vi "Read Voltage.vi"(6 "错误输入":cluster{"状态":bool, "代码":i32, "源":string}) -> (0 "错误输出":cluster{"状态":bool, "代码":i32, "源":string}, 3 "电压":dbl)   [LabVIEW 2012]
doc: "该VI用于LabVIEW核心课程I、II。\n\n该VI可模拟从DAQ板卡获取电压读数。在本课程中，该VI可代替温度读数相关练习中的“DAQ助手”Express VI。该VI可作为所有（演示）练习中的子VI使用。"
panel:
  # "该VI可用于演示读取设备1上通道0的电压值。该值调整100倍后转换为温度值。"
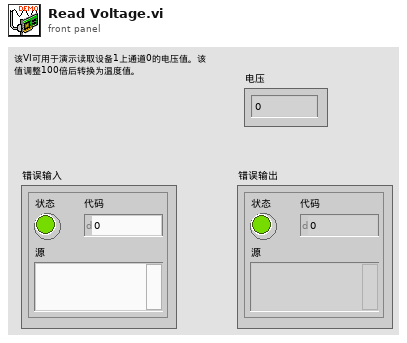
[diagram p1: front panel]
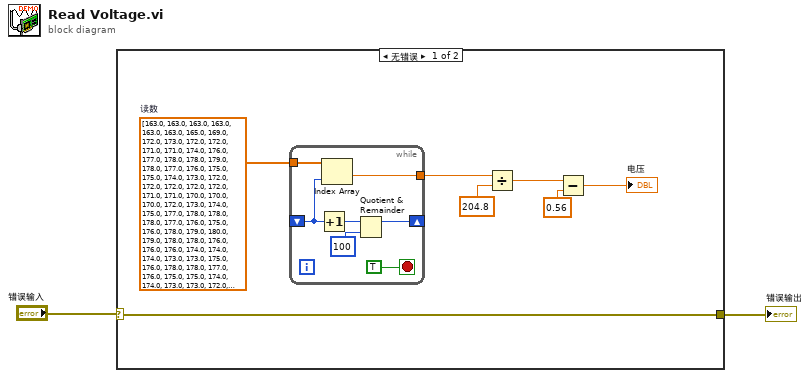
[diagram p0: block diagram]
diagram:
  n1 = case shown="无错误" "错误输入" {
    selector: "错误输入" -> [w5 w17]
    tunnel: [w5 w17] -> w2
    frame No Error {
      w3 = dbl[] [163.0, 163.0, 163.0, 163.0, 163.0, 163.0, 165.0, 169.0, 172.0, 173.0, 172.0, 172.0, 171.0, 171.0, 174.0, 176.0, 177.0, 178.0, 178.0, 179.0, 178.0, 177.0, 176.0, 175.0, 175.0, 174.0, 173.0, 172.0, 172.0, 172.0, 172.0, 172.0, 171.0, 171.0, 170.0, 170.0, 170.0, 172.0, 173.0, 174.0, 175.0, 177.0, 178.0, 178.0, 178.0, 177.0, 176.0, 175.0, 176.0, 178.0, 179.0, 180.0, 179.0, 178.0, 178.0, 176.0, 176.0, 176.0, 174.0, 174.0, 174.0, 173.0, 173.0, 175.0, 176.0, 178.0, 178.0, 177.0, 176.0, 175.0, 175.0, 174.0, 174.0, 173.0, 173.0, 172.0, 172.0, 171.0, 171.0, 170.0, 170.0, 170.0, 170.0, 170.0, 170.0, 170.0, 169.0, 166.0, 167.0, 169.0, 170.0, 169.0, 168.0, 168.0, 168.0, 168.0, 167.0, 167.0, 167.0, 167.0]  # 读数
      n2 = while {
        tunnel: w3 -> [w11]
        tunnel: [w12] -> w8
        shift-left: _ -> [w16]
        shift-right: [w13] -> _
        stop <- TRUE stop-if-true
        n3 = Increment ("加1")(x=w16) -> (x+1=w15:i32)
        n4 = Index Array ("索引数组")(array=w11, index=w16) -> (element=w12:dbl)
        n5 = Quotient & Remainder ("商与余数")(x=w15, y=100) -> (x-y*floor(x/y)=w13:i32)  [unwired: 1 out]
      }
      n6 = Divide ("除")(x=w8, y=204.8) -> (x/y=w7:dbl)
      n7 = Subtract ("减")(x=w7, y=0.56) -> (x-y=→"电压":dbl)
    }
    frame Error {
    }
  }
  "错误输出" <- w2
